vi "oopAPI_RX (SAP)_2.vi"(10 "port":u32=1, 11 "board":u32) -> (0 "error out":errorcluster)   [LabVIEW 2020]
uses:
  src/AIM664LV.lvlib
  src/_polimorphicInstances/session/Fdx Close Session (Port).vi
  <extravilib>/ChannelInstances/Tag-bool.lvlib
  <vilib>/platform/TimedLoop/XDataNode/XDataNode.xnode
  <vilib>/Platform/TimedLoop/XDataNode/nitl_modes.ctl
  <vilib>/Platform/TimedLoop/XDataNode/XDNodeRunTimeDep.lvlib
  <vilib>/Platform/TimedLoop/XDataNode/wakeup.ctl
  <vilib>/Platform/TimedLoop/XDataNode/timing_clust.ctl
  src/_polimorphicInstances/udpPort/Fdx Create Udp Port (RX-SAP).vi
  src/bsp/AFDX_Receive/Fdx Create Rx VL.vi
  src/_polimorphicInstances/session/Fdx Create Session (Rx-VL-Oriented).vi
  src/_polimorphicInstances/control/Fdx Start (Rx).vi
  src/_controls/comm_computedMAC-IP.ctl
  src/_controls/sap_config_rx.ctl
  src/_controls/comm_verification_rx.ctl
panel:
  out "MsgCount":u32
  out "MsgErrorCount":u32
  out "Duplicated":bool
  in  "VL Config":T1={"VlId"=0, "VLRange"=0, "VerificationMode"=0, "Bag"=0, "Jitter"=0, "MaxFrameLength"=0, "MaxSkew"=0, "VLBufSize"=32768, "FilterMode"=0, "FilterPosition"=0, "Padding"=0, "FilterMask"=0, "FilterData"=0, "MinFrameLength"=0} {"FilterMode" items=["FDX_RX_VL_FLT_DIS", "FDX_RX_VL_FLT_ENA ", "FDX_RX_VL_FLT_ENA_INV"]; "MaxFrameLength" format="%.0x"; "VerificationMode" items=["FDX_RX_VL_CHECK_ENA_DEFAULT"=65535, "FDX_RX_VL_CHECK_REDMAM"=16, "DX_RX_VL_CHECK_TRAFIC"=8, "FDX_RX_VL_CHECK_FRAMESIZE"=4, "FDX_RX_VL_CHECK_SNINTEG"=2, "FDX_RX_VL_CHECK_INVPAC"=1, "FDX_RX_VL_CHECK_DISA"=0]}
  in  "SapPort Config":T2
  out "FramesPerSecond":u32[](array[numeric])
  out "BytesPerSecond":u32[](array[numeric])
  out "src info":cluster{"ip src":u32, "udp src port":u32}
  in  "Processor":i32=-2
  in  "Period uS":i64=2000
  out "msg to read":u32
  in  "MsgCount(1)":u32=1
  in  "DefaultPayloadMode (Full)":u32(ring) items=["FDX_PAYLOAD_FULL", "FDX_PAYLOAD_IP_EXT", "FDX_PAYLOAD_IP", "FDX_PAYLOAD_MAC"]
  out "read time uS":u32(graph)
  out "BytesRead":u32
  out "irig time":T3
  out "current time":timestamp
  out "current irig time":T4
  out "computedAddresses":T5 {"MACsrc" format="%.0x"}
  out "Data":u8[](array[numeric])=[1, 2, 3, 4, 0, 0, 0, 0, 0, 0, 0, 0, 0, 0, 0, 0, 0, 0, 0, 0, 0, 0, 0, 0, 0, 0, 0, 0, 0, 0, 0, 0, 0, 0, 0, 0, 0, 0, 0, 0, 0, 0, 0, 0, 0, 0, 0, 0, 0, 0, 0, 0, 0, 0, 0, 0, 0, 0, 0, 0, 0, 0, 0, 0, 0, 0, 0, 0, 0, 0, 0, 0, 0, 0, 0, 0, 0, 0, 0, 0, 0, 0, 0, 0, 0, 0, 0, 0, 0, 0, 0, 0, 0, 0, 0, 0, 0, 0, 0, 0] format="%.0x"
  in  "stop":bool
  out "PortInitOut":T6 {"PortConfig" items=["FDX_SINGLE", "FDX_REDUNDANT"]}
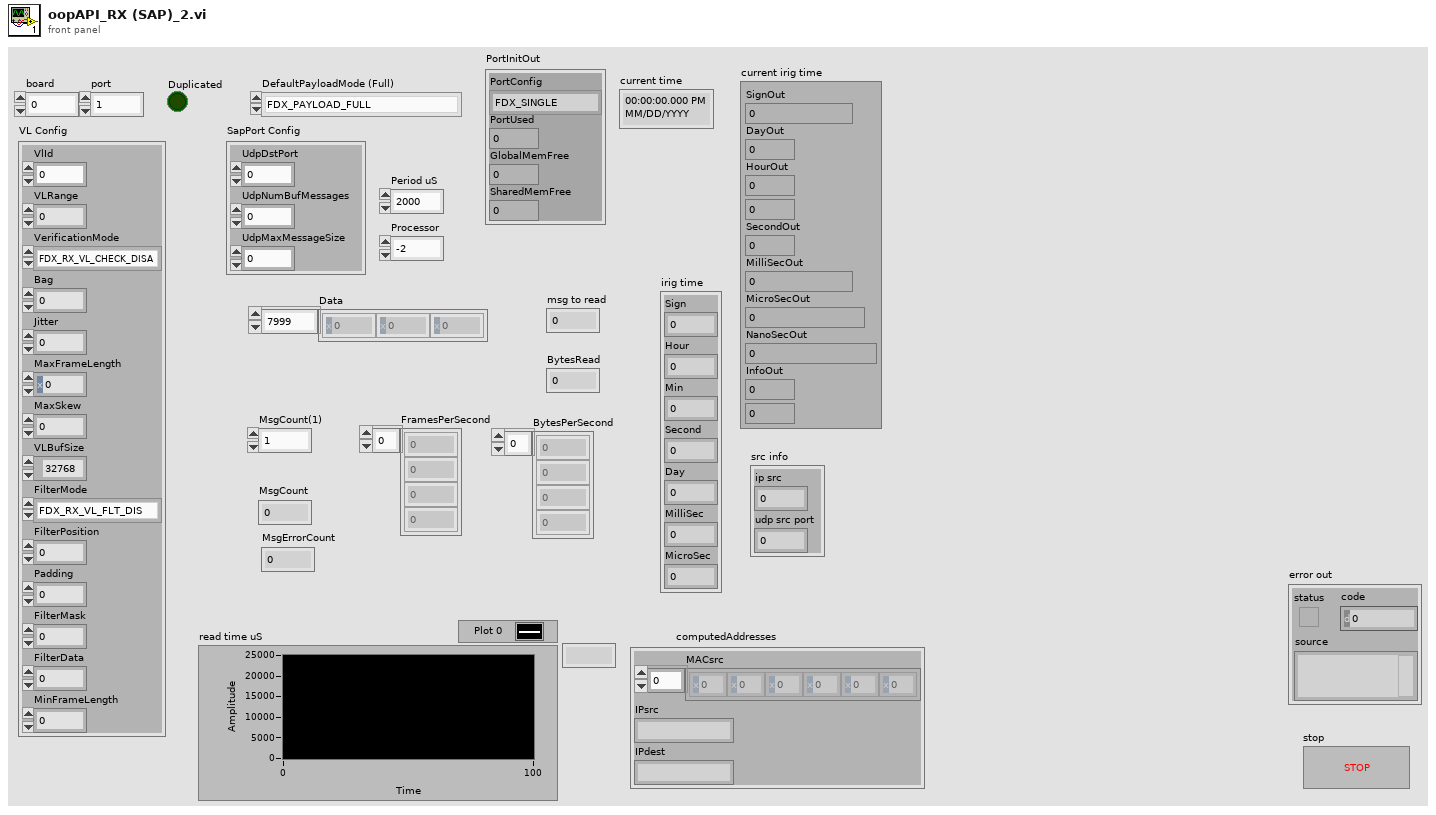
[diagram p1: front panel]
types:
  T1 = typedef "AIM664LV.lvlib/comm_verification_rx.ctl" = cluster{"VlId":u16, "VLRange":u32, "VerificationMode":u32, "Bag":u32, "Jitter":u32, "MaxFrameLength":u32, "MaxSkew":u32, "VLBufSize":u32, "FilterMode":u32, "FilterPosition":u32, "Padding":u32, "FilterMask":u32, "FilterData":u32, "MinFrameLength":u32}
  T2 = typedef "AIM664LV.lvlib/sap_config_rx.ctl" = cluster{"UdpDstPort":u16, "UdpNumBufMessages":u32, "UdpMaxMessageSize":u32}
  T3 = cluster{"Sign":i32, "Hour":u32, "Min":u32, "Second":u32, "Day":u32, "MilliSec":u32, "MicroSec":u32}
  T4 = cluster{"SignOut":i32, "DayOut":u32, "HourOut":u32, "MinOut":u32, "SecondOut":u32, "MilliSecOut":u32, "MicroSecOut":u32, "NanoSecOut":u32, "InfoOut":u32, "Mode":u32}
  T5 = typedef "AIM664LV.lvlib/comm_computedMAC-IP.ctl" = cluster{"MACsrc":u8[], "IPsrc":string, "IPdest":string}
  T6 = cluster{"PortConfig":u32, "PortUsed":u32, "GlobalMemFree":u32, "SharedMemFree":u32}
  T7 = typedef "XDNodeRunTimeDep.lvlib/timing_clust.ctl" = cluster{"Expected End [f-1]":u64, "Actual End [f-1]":u64, "Finished Late? [f-1]":bool, "Expected End [i-1]":u64, "Actual End [i-1]":u64, "Finished Late? [i-1]":bool, "Expected Start [i]":u64, "Actual Start [i]":u64, "Expected Start [f]":u64, "Actual Start [f]":u64, "Source Name":string, "Structure Name":string, "Period":i64, "Deadline":i64, "Offset":i64, "Start":i64, "Priority":i32, "Timeout":i32, "Mode":T8, "Wakeup Reason":T9, "Error":errorcluster, "Source Type":string, "Secondary Source Type":string, "Global End Time":u64, "Global Start Time":u64, "Frame Duration":u64, "Iteration Duration":u64, "Assigned CPU":i32, "I/O Scan Engine Mode":u32}
  T8 = typedef "XDNodeRunTimeDep.lvlib/nitl_modes.ctl" = enum32{"No Change", "Process missed periods, maintain original phase", "Discard missed periods, maintain original phase", "Process missed periods, ignore original phase", "Discard missed periods, ignore original phase"}
  T9 = typedef "XDNodeRunTimeDep.lvlib/wakeup.ctl" = enum32{"Normal", "Aborted", "Asynchronous wakeup", "Timing source error", "Timed loop error", "Timeout"}
  T10 = cluster{"TotalByteCount":u32[], "FrameGoodCount":u32[], "FrameErrorCount":u32[], "BytesPerSecond":u32[], "FramesPerSecond":u32[], "PhysErrorCount":u32[], "PreamErrorCount":u32[], "UnaligErrorCount":u32[], "CRCErrorCount":u32[], "IFGErrorCount":u32[], "IPErrorCount":u32[], "MACErrorCount":u32[], "NoSfdErrorCount":u32[], "VLLenErrorCount":u32[], "SNIntegrityErrorCount":u32[], "TrafShapingViolationCount":u32[], "MAC1Short":u32[], "MAC64To127Count":u32[], "MAC128To255Count":u32[], "MAC256To511Count":u32[], "MAC512To1023Count":u32[], "MAC1024To1518Count":u32[], "MACLong":u32[]}
  T11 = typedef "Tag-bool.lvlib/))Channel.ctl" = refnum<queue>
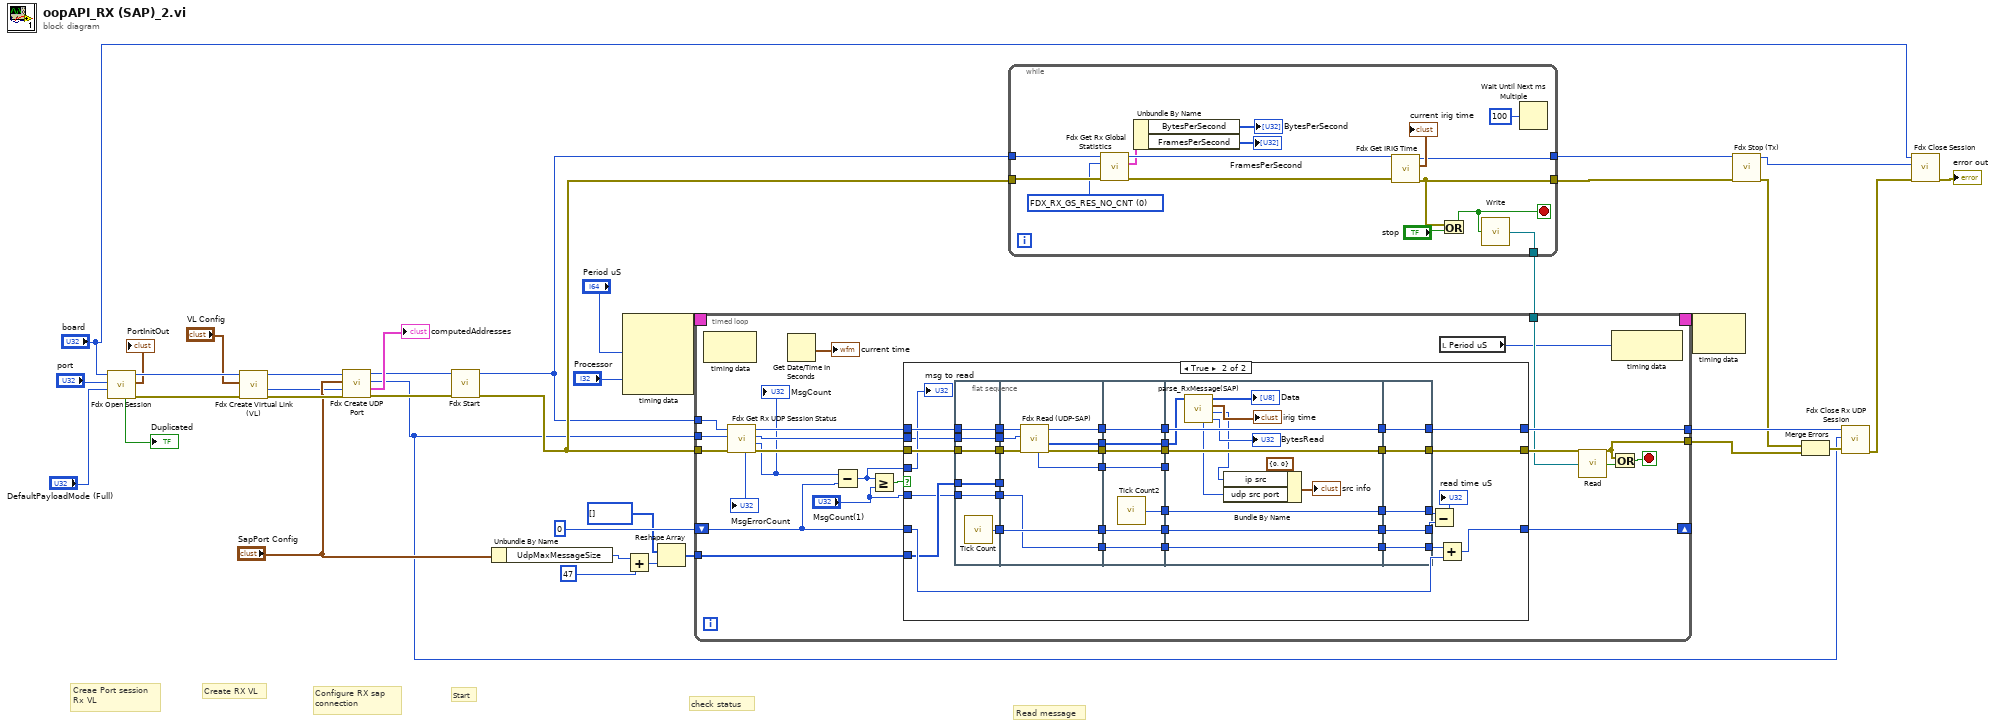
[diagram p0: block diagram]
diagram:
  # "Read message"
  # "check status"
  # "Start"
  # "Configure RX sap \nconnection"
  # "Create RX VL"
  # "Creae Port session\nRx VL"
  n1 = call-poly "Fdx Open Session.vi"("DefaultPayloadMode (Full)"="DefaultPayloadMode (Full)", "port"="port", "board"="board") -> ("error out"=w10:errorcluster, "PortInitOut"=→"PortInitOut":T6, "InstrumentHandle_port out"=w33:u32, "Duplicated"=→"Duplicated":bool)  [unwired: 3 in, 2 out]
  n2 = call-poly "Fdx Create Virtual Link (VL).vi"("error in (no error)"=w10, "VL Config"="VL Config", "InstrumentHandle_port in"=w33) -> ("error out"=w11:errorcluster, "VlId"=w5:u16, "InstrumentHandle_port out"=w12:u32)  [unwired: 6 in]
  n3 = call-poly "Fdx Create UDP Port.vi"("error in (no error)"=w11, "VlId"=w5, "SapPort Config"="SapPort Config", "port handle in"=w12) -> ("error out"=w37:errorcluster, "computedAddresses"=→"computedAddresses":T5, "sapPort handle out"=w3:u32, "port handle out"=w35:u32)  [unwired: 4 in]
  n4 = call-poly "Fdx Start.vi"("error in (no error)"=w37, "InstrumentHandle_port in"=w35) -> ("error out"=w29:errorcluster, "InstrumentHandle_port out"=w4:u32)  [unwired: 8 in]
  n5 = Unbundle By Name("SapPort Config") -> ("UdpMaxMessageSize"=w8:u32)
  n6 = node-c288("Period uS", "Processor") -> (w20:T7)  [unwired: 2 in]
  n7 = Add(x=w8, y=u32 47) -> (x+y=w15:u32)
  n8 = Reshape Array(u8[] [] ("Buffer In"), w15) -> (w13:u8[])
  n9 = while {
    tunnel: w4 -> [w52]
    tunnel: w29 -> [w44]
    tunnel: [w50] -> w28
    tunnel: [w49] -> w27
    tunnel: [w47] -> w25
    stop <- w48 stop-if-true
    w39 = u32 0 items=["FDX_RX_GS_RES_NO_CNT", "FDX_RX_GS_RES_ALL_CNT", "FDX_RX_GS_RES_ERR_CNT"] ("Control")
    n10 = call "Fdx Get Rx Global Statistics.vi"("error in (no error)"=w44, "Control"=w39, "InstrumentHandle_port in"=w52) -> ("error out"=w43:errorcluster, "GlobalStat Out"=w42:T10, "InstrumentHandle_port out"=w45:u32)  [unwired: 6 in]
    n11 = Unbundle By Name(w42) -> ("BytesPerSecond"=→"BytesPerSecond":u32[], "FramesPerSecond"=→"FramesPerSecond":u32[])
    n12 = call "Fdx Get IRIG Time.vi"("error in (no error)"=w43, "InstrumentHandle_board in"=w45) -> ("error out"=w49:errorcluster, "Curent Irig Time"=→"current irig time":T4, "InstrumentHandle_board out"=w50:u32)  [unwired: 7 in]
    n13 = Or(x=w49, y="stop") -> (x .or. y?=w48:bool)
    n14 = call <extravilib>:"Write.vi"("element"=w48) -> ("channel"=w47:T11)  [unwired: 1 out]
    n15 = Wait Until Next ms Multiple(millisecond multiple=u32 100) -> ()  [unwired: 1 out]
  }
  n16 = timed-loop {
    tunnel: w29 -> [w68]
    tunnel: w3 -> [w58]
    tunnel: [w72] -> w30
    tunnel: [w71] -> w22
    tunnel: w25 -> [w69]
    shift-right: [w62] -> _
    shift-left: 0 -> [w64]
    timing: w20 -> [_]
    timing-out: [_] -> w19
    tunnel: w13 -> [w59]
    tunnel: w4 -> [w57]
    stop <- w74 stop-if-true
    n17 = node-c288() -> ()  [unwired: 1 in, 1 out]
    n18 = call "Fdx Get Rx UDP Session Status.vi"("error in (no error)"=w68, "UdpHandle in"=w58, "InstrumentHandle_port in"=w57) -> ("error out"=w66:errorcluster, "MsgCount"=w55:u32, "UdpHandle out"=w56:u32, "InstrumentHandle_port out"=w67:u32, "MsgErrorCount"=→"MsgErrorCount":u32)  [unwired: 4 in]
    "MsgCount" <- w55
    n19 = Get Date/Time In Seconds() -> (seconds since 1Jan1904=→"current time":timestamp)
    n20 = Subtract(x=w55, y=w64) -> (x-y=w61:u32)
    n21 = Greater Or Equal?(x=w61, y="MsgCount(1)") -> (x >= y?=w65:bool)
    n22 = case shown="True" w65 {
      tunnel: w66 -> [w80 w101]
      tunnel: w67 -> [w81 w100]
      tunnel: [w81 w96] -> w72
      tunnel: [w80 w95] -> w71
      tunnel: "MsgCount(1)" -> [_ w84]
      tunnel: w64 -> [w79 w90]
      tunnel: [w79 w89] -> w62
      tunnel: w61 -> [_ w88]
      tunnel: w59 -> [_ w86]
      tunnel: w56 -> [_ w82]
      frame False {
      }
      frame True {
        n23 = flat-sequence {
          tunnel: w101 -> [w124]
          tunnel: w100 -> [w125]
          tunnel: [w125] -> w119
          tunnel: [w124] -> w118
          tunnel: [w123] -> w117
          tunnel: [w122] -> w87
          tunnel: w86 -> [w122]
          tunnel: [w121] -> w85
          tunnel: w84 -> [w121]
          tunnel: [w120] -> w83
          tunnel: w82 -> [w120]
          tunnel: w119 -> [w129]
          tunnel: w118 -> [w130]
          tunnel: w117 -> [w134]
          tunnel: [w134] -> w116
          tunnel: [w133] -> w115
          tunnel: [w132] -> w114
          tunnel: [w131] -> w113
          tunnel: [w128] -> w112
          tunnel: [w127] -> w92
          tunnel: w87 -> [_]
          tunnel: w85 -> [w127]
          tunnel: w83 -> [w126]
          tunnel: w116 -> [w141]
          tunnel: [w141] -> w111
          tunnel: [w140] -> w110
          tunnel: [w139] -> w109
          tunnel: w115 -> [w139]
          tunnel: [w138] -> w108
          tunnel: w114 -> [w138]
          tunnel: [w137] -> w107
          tunnel: w113 -> [w137]
          tunnel: [w136] -> w106
          tunnel: w112 -> [w136]
          tunnel: [w135] -> w93
          tunnel: w92 -> [w135]
          tunnel: w111 -> [w154]
          tunnel: [w154] -> w105
          tunnel: [w153] -> w104
          tunnel: w110 -> [w153]
          tunnel: [w152] -> w103
          tunnel: w109 -> [w152]
          tunnel: [w151] -> w102
          tunnel: w108 -> [w151]
          tunnel: w107 -> [w149]
          tunnel: w106 -> [_]
          tunnel: [w150] -> w94
          tunnel: w93 -> [w150]
          tunnel: [w159] -> w99
          tunnel: w105 -> [w159]
          tunnel: [w158] -> w97
          tunnel: w104 -> [w158]
          tunnel: [w157] -> w96
          tunnel: w103 -> [w157]
          tunnel: [w156] -> w95
          tunnel: w102 -> [w156]
          tunnel: [w155] -> w91
          tunnel: w94 -> [w155]
          frame #0 {
            n24 = call "Tick Count"() -> ("Tick Count(uSec)"=w123:u32)
          }
          frame #1 {
            n25 = call "Fdx Read (UDP-SAP).vi"("error in"=w130, "UdpHandle in"=w126, "InstrumentHandle_port in"=w129) -> ("error out"=w132:errorcluster, "Data"=w131:u8[], "InstrumentHandle_port out"=w133:u32, "MsgRead"=w128:u32)  [unwired: 4 in, 1 out]
          }
          frame #2 {
            n26 = call "Tick Count2"() -> ("Tick Count(uSec)"=w140:u32)
          }
          frame #3 {
            n27 = call "parse_RxMessage(SAP).vi"("ReadBuffer In"=w149) -> ("msg size"=→"BytesRead":u32, "ip src"=w142:u32, "IrigTime"=→"irig time":T3, "Message Data"=→"Data":u8[], "udp src port"=w143:u32)  [unwired: 6 in]
            n28 = Bundle By Name(cluster=cluster{"ip src":u32, "udp src port":u32} {"ip src"=0, "udp src port"=0} ("src info"), "ip src"=w142, "udp src port"=w143) -> (→"src info":cluster{"ip src":u32, "udp src port":u32})
          }
          frame #4 {
          }
        }
        n29 = Subtract(x=w97, y=w99) -> (x-y=→"read time uS":u32)
        n30 = Add(x=w91, y=w90) -> (x+y=w89:u32)
        "msg to read" <- w88
      }
    }
    n31 = local read "Period uS"() -> (w60:i64)
    n32 = call <extravilib>:"Read.vi"("channel"=w69) -> ("element"=w70:bool)  [unwired: 1 in, 1 out]
    n33 = node-c288(w60) -> ()  [unwired: 1 out]
    n34 = Or(x=w71, y=w70) -> (x .or. y?=w74:bool)
  }
  n35 = node-c288(w19) -> ()  [unwired: 1 out]
  n36 = call "Fdx Stop (Tx).vi"("error in (no error)"=w27, "InstrumentHandle_port in"=w28) -> ("error out"=w23:errorcluster, "InstrumentHandle_port out"=w1:u32)  [unwired: 8 in]
  n37 = Merge Errors(w23, w22) -> (w24:errorcluster)
  n38 = call "Fdx Close Rx UDP Session.vi"("error in (no error)"=w24, "UdpHandle in"=w3, "InstrumentHandle_port in"=w30) -> ("error out"=w26:errorcluster)  [unwired: 7 in, 1 out]
  n39 = call-poly "Fdx Close Session.vi"("error in (no error)"=w26, "InstrumentHandle_port in"=w1, "InstrumentHandle_board in"="board") -> ("error out"=→"error out":errorcluster)  [unwired: 8 in]
